vi "StartIndex.vi"(0 "Axis In (Axis Space)":T1=enum."Axis Space", 11 "error in (no error)":errorcluster) -> (4 "Axis Out":T1, 15 "error out":errorcluster)   [LabVIEW 2009]
doc: "Start the Index specified by the Host Index parameter currently set on the axis. If the drive is disabled, function does nothing."
uses:
  typedefs/AxisSelect_Enum.ctl
  typedefs/Ultra3000/Func.ctl
  typedefs/Ultra3000/Cmds.ctl
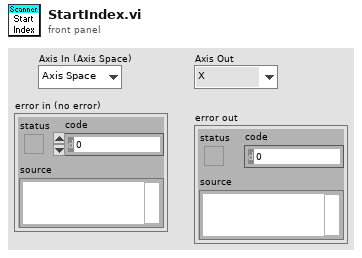
[diagram p1: front panel]
types:
  T1 = typedef "AxisSelect_Enum.ctl" = enum16{"X", "Y", "Z", "Axis Space"}
  T2 = typedef "DriveStatus_Cluster.ctl" = cluster{"In-position":bool, "Zero Speed":bool, "Enabled":bool, "Fault Disable":bool, "Ready":bool, "Start Index":bool, "Overtravel Exceeded":bool, "Up to Speed":bool, "Sequence Complete":bool}
  T3 = typedef "Func.ctl" = u16
  T4 = typedef "Cmds.ctl" = u16
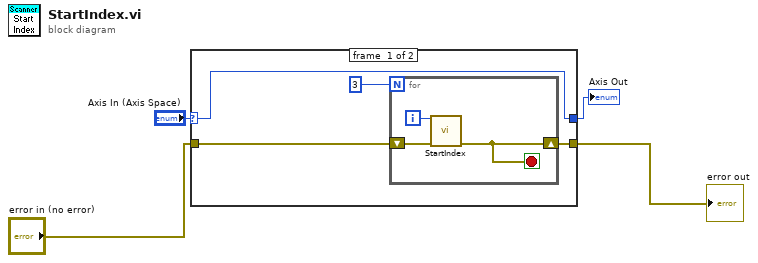
[diagram p0: block diagram]
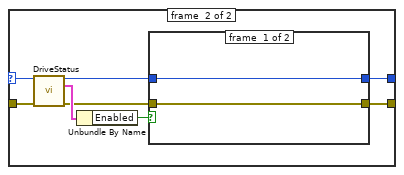
[diagram p2: hidden frame]
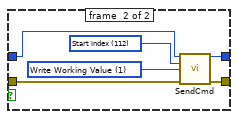
[diagram p3: hidden frame]
diagram:
  n1 = case shown="\"X\"..\"Z\"" "Axis In (Axis Space)" {
    selector: "Axis In (Axis Space)" -> [w7 w15]
    tunnel: [w5 w14] -> w2
    tunnel: [w7 w13] -> w3
    tunnel: "error in (no error)" -> [w6 w12]
    frame #0 {
      n2 = for {
        N: 3 -> [_]
        shift-right: [w9] -> w5
        shift-left: w6 -> [w10]
        i -> [w11]
        stop <- w9 stop-if-true
        n3 = call "StartIndex.vi"("Axis In (Axis Space)"=w11, "error in (no error)"=w10) -> ("error out"=w9:errorcluster)  [unwired: 12 in, 1 out]
      }
    }
    frame #1 {
      n4 = call "DriveStatus.vi"("Axis In"=w15, "error in (no error)"=w12) -> ("Axis Out"=w16:T1, "Status"=w19:T2, "error out"=w17:errorcluster)  [unwired: 11 in]
      n5 = Unbundle By Name(w19) -> ("Enabled"=w18:bool)
      n6 = case shown="True" w18 {
        tunnel: [w21 w27] -> w13
        tunnel: [w20 w26] -> w14
        tunnel: w16 -> [w21 w23]
        tunnel: w17 -> [w20 w22]
        frame #0 {
        }
        frame #1 {
          w25 = T3 1 items=["Read Working Value", "Write Working Value", "Read Non-Volatile Value", "Write Non-Volatile and Woring Value", "Copy Non-Volatile Value to Working Value", "Copy Working Value to Non-Volatile Value", "Read Default Value", "Copy Default Value to Non-Volatile and Working Values", "Read Min Value", "Read Max Value", "Read Array Index Min", "Read Array Index Max"] ("Function")
          w24 = T4 112 items=["Position Command"=128, "Run Status"=117, "Fault Status"=116, "Position Error"=129, "Auto-Start Homing"=196, "Start Homing"=205, "Homing Type"=197, "Motor Position"=126, "Velocity Motor"=133, "Power-Up Status"=1, "Drive Name"=6, "Position Window Size"=22, "Position Window Time"=23, "Zero Speed Limit"=34, "Speed Window Size"=35, "Up to Speed Limit"=37, "Forward Current Limit"=47, "Reverse Current Limit"=48, "Override Mode"=67, "Operation Mode"=90, "Host Control Mode"=97, "Reset Drive"=106, "Drive Enable"=107, "Setpoint Current"=108, "Setpoint Velocity"=109, "Setpoint Acceleration"=110, "Reset Faults"=111, "Position Comparator"=349, "Postition Comparator Polarity"=350, "Position Rollover Enable"=404, "Baud Rate"=80, "Frame Format"=81, "Drive Address"=82, "Broadcast Address"=83, "Auto-start Indexing"=88, "Start Index"=112, "Host Index"=184, "Index Type"=174, "Index Dist/Pos"=175, "Index Reg Dist"=176, "Index Velocity"=177, "Index Acceleration"=178, "Index Deceleration"=179, "Index Dwell"=180, "Index Count"=181, "Index Termination"=182, "Index Pointer"=183, "Index Abort Deceleration"=185, "Positive Soft Pos Limit"=216, "Define Home"=113, "Negative Soft Pos Limit"=217] ("Command")
          n7 = call "SendCmd.vi"("Axis In"=w23, "Command"=w24, "Function"=w25, "error in (no error)"=w22) -> ("Axis Out"=w27:T1, "error out"=w26:errorcluster)  [unwired: 8 in, 2 out]
        }
      }
    }
  }
  "Axis Out" <- w3
  "error out" <- w2
